vi "ReadOrSaveCases.vi"(9 "Location":enum16{"CUMC", "SERI", "VMR", "Aline", "UTEX"}(ring)=enum."SERI", 10 "New Case":T1, 11 "Save(T)\\Read(F)":bool) -> (2 "Case List":string[](array[string]), 3 "CaseArray":T2(array[cluster]))   [LabVIEW 2022 SP3]
uses:
  ScanningControl/Digitizers/-DigitizerRoutines/Digitizer.ctl
panel:
  out "path":path
  in  "Acquistion Parameters":T3={"Sampling Rate"=250.0, "Ref Delay (ms)"=0.0, "rf points per line"=2048, "rf lines"=256, "Dig Scale"=4.0} {"Dig Scale" items=["5 V"=5.0, "2 V"=2.0, "1 V"=1.0, "500 mV"=0.5, "200 mV"=0.2, "100 mV"=0.1, "50 mV"=0.05]; "rf lines" min=1; "rf points per line" min=1; "Ref Delay (ms)" format="%.2f"}
  in  "Sector?":bool=TRUE
  in  "Filter Prams":T4={"low cutoff"=20, "order"=81, "high cutoff"=60}
  in  "Timeout (s)":dbl=0.15
  in  "Probe":T5(ring)
  in  "Scan Info":T6
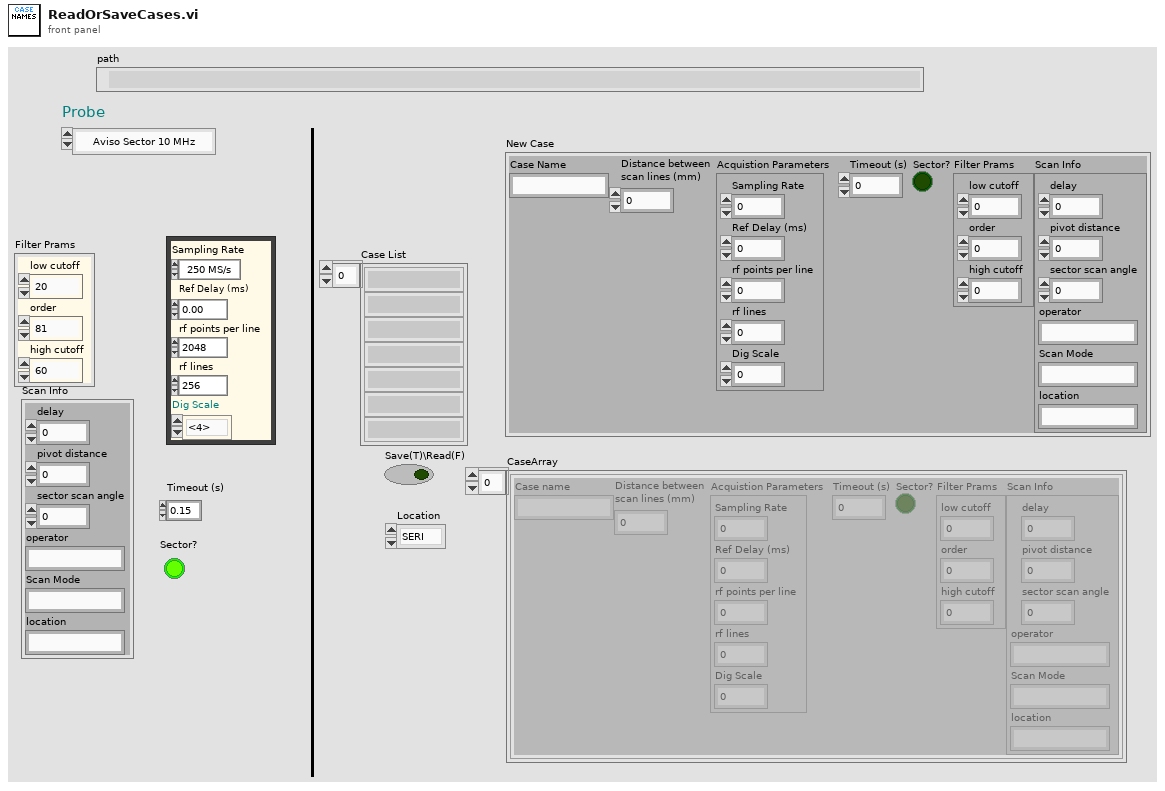
[diagram p1: front panel]
types:
  T1 = cluster{"Case Name":string, "Distance between\nscan lines (mm)":sgl, "Acquistion Parameters":cluster{"Sampling Rate":dbl, "Ref Delay (ms)":dbl, "rf points per line":i32, "rf lines":i32, "Dig Scale":dbl}, "Timeout (s)":dbl, "Sector?":bool, "Filter Prams":cluster{"low cutoff":i32, "order":i32, "high cutoff":i32}, "Scan Info":cluster{"delay":sgl, "pivot distance":sgl, "sector scan angle":sgl, "operator":string, "Scan Mode":string, "location":string}}
  T2 = cluster{"Case name":string, "Distance between\nscan lines (mm)":sgl, "Acquistion Parameters":cluster{"Sampling Rate":dbl, "Ref Delay (ms)":dbl, "rf points per line":i32, "rf lines":i32, "Dig Scale":dbl}, "Timeout (s)":dbl, "Sector?":bool, "Filter Prams":cluster{"low cutoff":i32, "order":i32, "high cutoff":i32}, "Scan Info":cluster{"delay":sgl, "pivot distance":sgl, "sector scan angle":sgl, "operator":string, "Scan Mode":string, "location":string}}[]
  T3 = cluster{"Sampling Rate":dbl, "Ref Delay (ms)":dbl, "rf points per line":i32, "rf lines":i32, "Dig Scale":dbl}
  T4 = cluster{"low cutoff":i32, "order":i32, "high cutoff":i32}
  T5 = enum16{"Aviso Sector 10 MHz", "Aviso Sector 20 MHz Retina", "Aviso Sector 20 MHz", "Aviso Lin50", "UTEX 50MHz", "Custom"}
  T6 = cluster{"delay":sgl, "pivot distance":sgl, "sector scan angle":sgl, "operator":string, "Scan Mode":string, "location":string}
  T7 = typedef "Digitizer.ctl" = enum16{"Acqiris Digitizer", "NI Digitizer", "LeCroy", "GaGe", "AlazarTech", "No Digitizer", "Teledyne"}
  T8 = enum16{"open", "replace", "create", "open or create", "replace or create", "replace or create with confirmation"}
  T9 = cluster{"Case Name":string, "Distance between\nscan lines (mm)":sgl, "Acquistion Parameters":cluster{"Sampling Rate":dbl, "Ref Delay (ms)":dbl, "rf points per line":i32, "rf lines":i32, "Dig Scale":dbl}, "Timeout (s)":dbl, "Sector?":bool, "Filter Prams":cluster{"low cutoff":i32, "order":i32, "high cutoff":i32}, "Scan Info":cluster{"delay":sgl, "pivot distance":sgl, "sector scan angle":sgl, "operator":string, "Scan Mode":string, "location":string}}[]
  T10 = cluster{"Sampling Rate":dbl, "Ref Delay (ms)":dbl, "rf points per line":i32, "rf lines":i32, "Voltage Scale 1":dbl}
  T11 = enum16{"Aviso Sector 10 MHz", "Aviso Sector 20 MHz Retina", "Aviso Sector 20 MHz", "Aviso Lin50", "Custom"}
  T12 = cluster{string, "Distance between\nscan lines (mm)":sgl, "Acquistion Parameters":cluster{"Sampling Rate":dbl, "Ref Delay (ms)":dbl, "rf points per line":i32, "rf lines":i32, "Dig Scale":dbl}, "Timeout (s)":dbl, "Sector?":bool, "Filter Prams":cluster{"low cutoff":i32, "order":i32, "high cutoff":i32}, "Scan Info":cluster{"delay":sgl, "pivot distance":sgl, "sector scan angle":sgl, "operator":string, "Scan Mode":string, "location":string}}
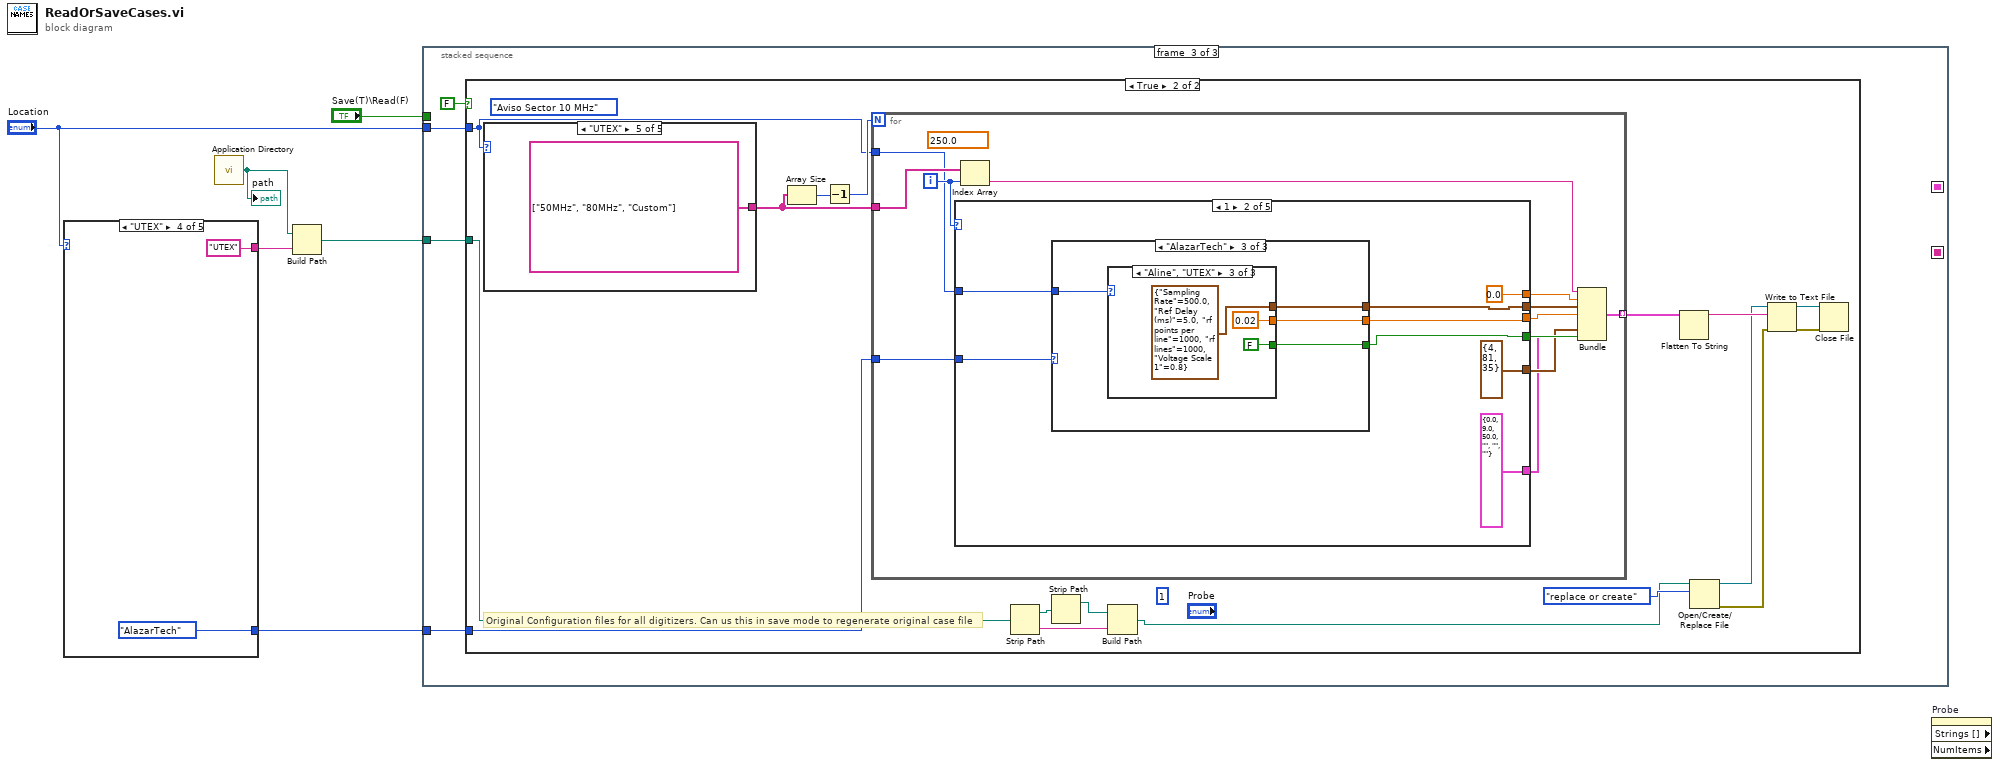
[diagram p0: block diagram]
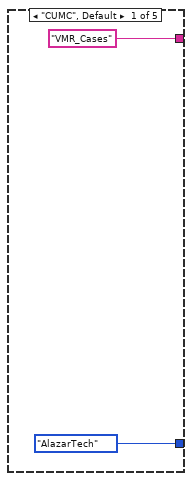
[diagram p2: hidden frame]
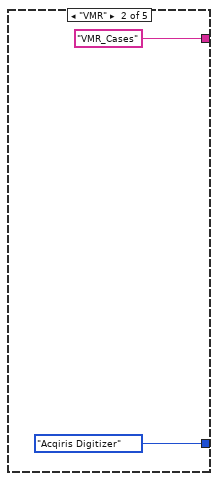
[diagram p3: hidden frame]
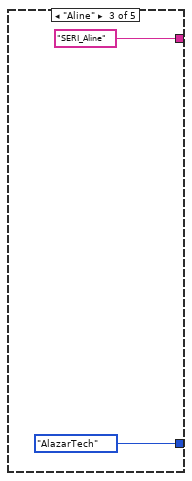
[diagram p4: hidden frame]
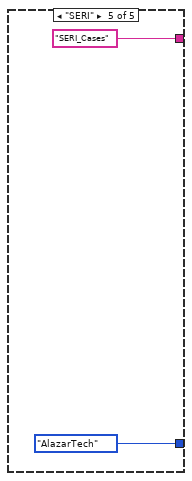
[diagram p5: hidden frame]
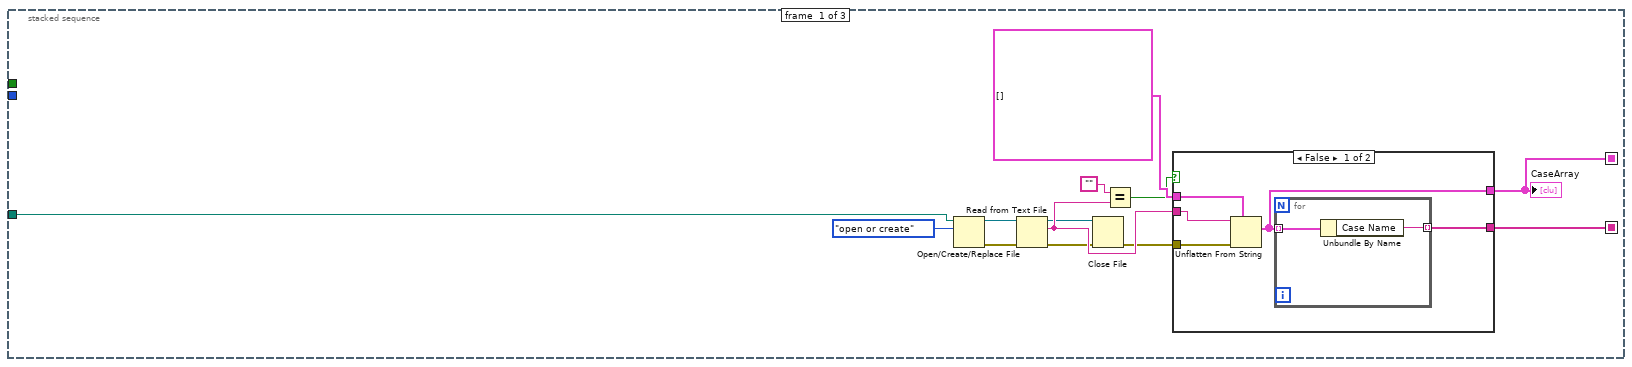
[diagram p6: hidden frame]
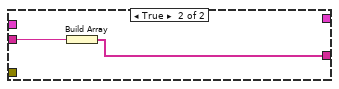
[diagram p7: hidden frame]
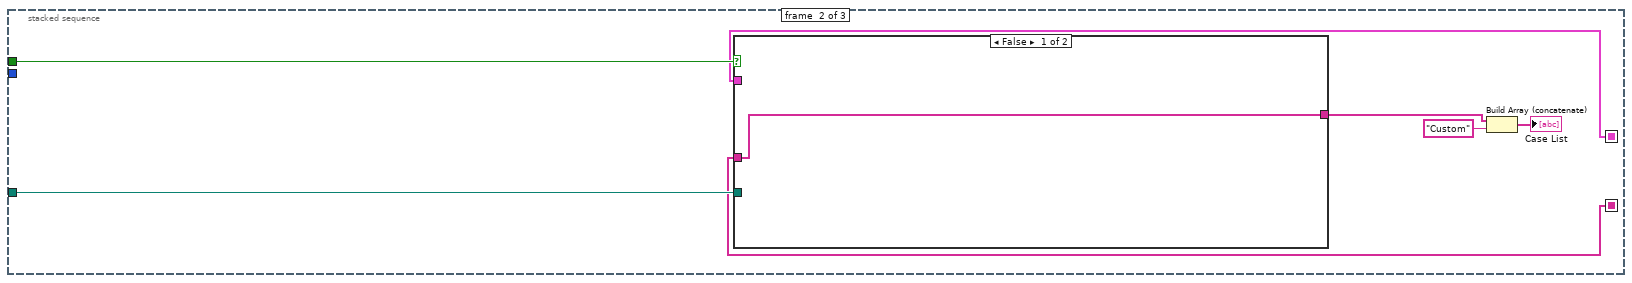
[diagram p8: hidden frame]
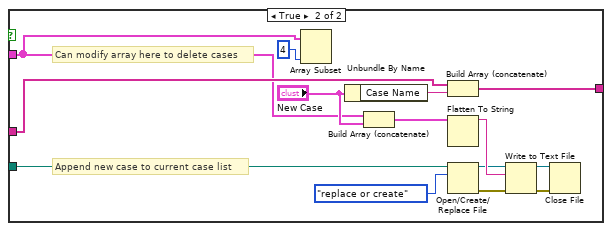
[diagram p9: hidden frame]
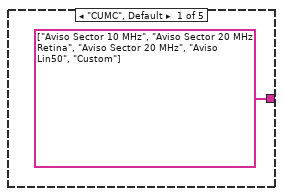
[diagram p11: hidden frame]
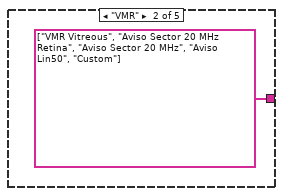
[diagram p12: hidden frame]
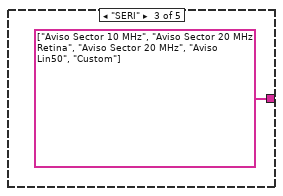
[diagram p13: hidden frame]
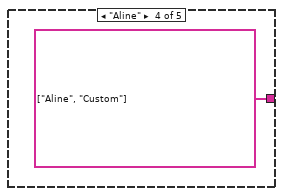
[diagram p14: hidden frame]
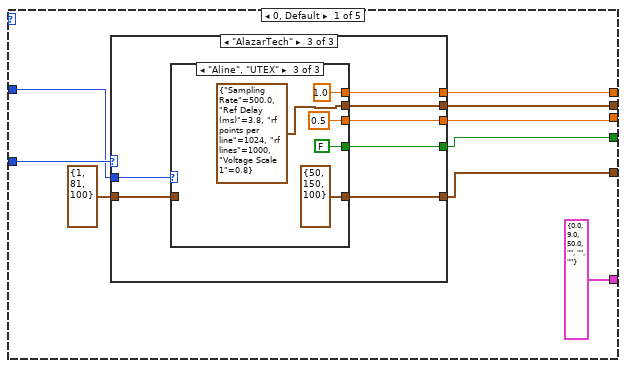
[diagram p15: hidden frame]
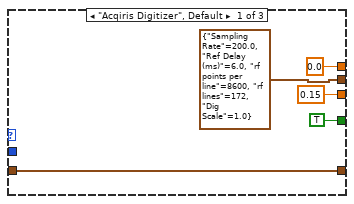
[diagram p16: hidden frame]
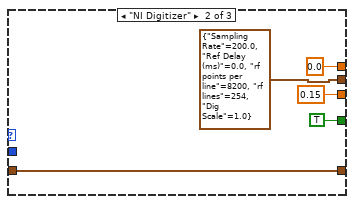
[diagram p17: hidden frame]
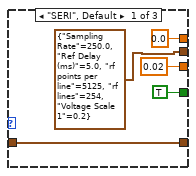
[diagram p18: hidden frame]
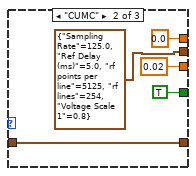
[diagram p19: hidden frame]
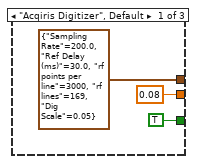
[diagram p20: hidden frame]
diagram:
  n1 = case shown="\"UTEX\"" "Location" {
    tunnel: ["VMR_Cases" "VMR_Cases" "SERI_Aline" "UTEX" "SERI_Cases"] -> w4
    tunnel: [Digitizer."AlazarTech" ("Main Digitizer") Digitizer."Acqiris Digitizer" ("Main Digitizer") Digitizer."AlazarTech" ("Main Digitizer") Digitizer."AlazarTech" ("Main Digitizer") Digitizer."AlazarTech" ("Main Digitizer")] -> w1
    frame "CUMC", Default {
    }
    frame "VMR" {
    }
    frame "Aline" {
    }
    frame "UTEX" {
    }
    frame "SERI" {
    }
  }
  n2 = call <vilib>:"Application Directory.vi"() -> ("Application Directory"=w3:path)
  "path" <- w3
  n3 = Build Path(base path=w3, name or relative path=w4) -> (appended path=w5:path)
  n4 = stacked-sequence {
    seq-local: [w18 _ _] -> [_ w44 _]
    seq-local: [w17 _ _] -> [_ w42 _]
    tunnel: w5 -> [w28 w43 w64]
    tunnel: "Save(T)\\Read(F)" -> [_ w45 _]
    tunnel: "Location" -> [_ _ w63]
    tunnel: w1 -> [_ _ w61]
    frame #0 {
      n5 = Open/Create/Replace File(file path (use dialog)=w28, operation (0:open)=T8."open or create") -> (refnum out=w27:refnum<file>, error out=w26:errorcluster)  [unwired: 4 in, 1 out]
      n6 = Read from Text File(file (use dialog)=w27, error in=w26) -> (refnum out=w19:refnum<file>, text=w23:string, error out=w21:errorcluster)  [unwired: 2 in, 1 out]
      n7 = Close File(refnum=w19, error in=w21) -> (error out=w20:errorcluster)  [unwired: 1 out]
      n8 = Equal?(x="", y=w23) -> (x = y?=w22:bool)
      n9 = case shown="False" w22 {
        tunnel: T9 [] -> [w34 _]
        tunnel: w20 -> [w33 _]
        tunnel: w23 -> [w32 w38]
        tunnel: [w31 w37] -> w17
        tunnel: [w30 _] -> w18
        frame False {
          n10 = Unflatten From String(type=w34, binary string=w32, error in (no error)=w33) -> (value=w30:T9)  [unwired: 2 in, 2 out]
          n11 = for {
            tunnel: w30 -> [w36] mode=indexing
            tunnel: [w35] -> w31 mode=indexing
            n12 = Unbundle By Name(w36) -> ("Case Name"=w35:string)
          }
        }
        frame True {
          n13 = Build Array(w38) -> (w37:string[])
        }
      }
      "CaseArray" <- w18
    }
    frame #1 {
      n14 = case shown="False" w45 {
        tunnel: w44 -> [_ w49]
        tunnel: w43 -> [_ w54]
        tunnel: w42 -> [w46 w52]
        tunnel: [w46 w50] -> w41
        frame False {
        }
        frame True {
          # "Can modify array here to delete cases"
          # "Append new case to current case list"
          n15 = Array Subset(array=w49, length=4) -> ()  [unwired: 1 in, 1 out]
          n16 = Unbundle By Name("New Case") -> ("Case Name"=w51:string)
          n17 = Build Array (concatenate)(w49, "New Case") -> (w47:T9)
          n18 = Build Array (concatenate)(w52, w51) -> (w50:string[])
          n19 = Flatten To String(anything=w47) -> (data string=w60:string)  [unwired: 3 in, 2 out]
          n20 = Open/Create/Replace File(file path (use dialog)=w54, operation (0:open)=T8."replace or create") -> (refnum out=w56:refnum<file>, error out=w57:errorcluster)  [unwired: 4 in, 1 out]
          n21 = Write to Text File(file (use dialog)=w56, text=w60, error in=w57) -> (refnum out=w59:refnum<file>, error out=w58:errorcluster)  [unwired: 1 in, 1 out]
          n22 = Close File(refnum=w59, error in=w58) -> ()  [unwired: 2 out]
        }
      }
      n23 = Build Array (concatenate)(w41, "Custom" ("Case Name")) -> (→"Case List":string[])
    }
    frame #2 {
      n24 = case shown="True" FALSE {
        tunnel: w64 -> [_ w69]
        tunnel: w63 -> [_ w73]
        tunnel: w61 -> [_ w70]
        frame False {
        }
        frame True {
          (unwired) 1
          (unwired) T11."Aviso Sector 10 MHz" ("Probe")
          # "Original Configuration files for all digitizers. Can us this in save mode to regenerate original case file"
          n25 = case shown="\"UTEX\"" w73 {
            tunnel: [string[] ["Aviso Sector 10 MHz", "Aviso Sector 20 MHz Retina", "Aviso Sector 20 MHz", "Aviso Lin50", "Custom"] ("Strings []") string[] ["VMR Vitreous", "Aviso Sector 20 MHz Retina", "Aviso Sector 20 MHz", "Aviso Lin50", "Custom"] ("Strings []") string[] ["Aviso Sector 10 MHz", "Aviso Sector 20 MHz Retina", "Aviso Sector 20 MHz", "Aviso Lin50", "Custom"] ("Strings []") string[] ["Aline", "Custom"] ("Strings []") string[] ["50MHz", "80MHz", "Custom"] ("Strings []")] -> w72
            frame "CUMC", Default {
            }
            frame "VMR" {
            }
            frame "SERI" {
            }
            frame "Aline" {
            }
            frame "UTEX" {
            }
          }
          n26 = Array Size(array=w72) -> (size(s)=w71:i32)
          n27 = Decrement(x=w71) -> (x-1=w74:i32)
          n28 = for {
            N: w74 -> [_]
            tunnel: w72 -> [w89]
            tunnel: [w91] -> w79 mode=indexing
            tunnel: w73 -> [w88]
            tunnel: w70 -> [w87]
            i -> [w90]
            (unwired) 250.0 ("Sampling Rate")
            n29 = case shown="1" w90 {
              tunnel: [w101 sgl 0.0 sgl 0.0 sgl 50.0 sgl 0.0 ("Distance between\nscan lines (mm)")] -> w98
              tunnel: [w107 w146 w173 w191 "Acquistion Parameters"] -> w97
              tunnel: [w99 T4 {"low cutoff"=4, "order"=81, "high cutoff"=35} ("Filter Prams") T4 {"low cutoff"=4, "order"=81, "high cutoff"=35} ("Filter Prams") T4 {"low cutoff"=20, "order"=81, "high cutoff"=60} ("Filter Prams") "Filter Prams"] -> w94
              tunnel: [T6 {"delay"=0.0, "pivot distance"=9.0, "sector scan angle"=50.0, "operator"="", "Scan Mode"="", "location"=""} ("Scan Info") T6 {"delay"=0.0, "pivot distance"=9.0, "sector scan angle"=50.0, "operator"="", "Scan Mode"="", "location"=""} ("Scan Info") T6 {"delay"=0.0, "pivot distance"=9.0, "sector scan angle"=50.0, "operator"="", "Scan Mode"="", "location"=""} ("Scan Info") T6 {"delay"=0.0, "pivot distance"=0.0, "sector scan angle"=0.0, "operator"="", "Scan Mode"="", "location"=""} ("Scan Info") "Scan Info"] -> w93
              tunnel: w87 -> [w105 w143 w170 w192 _]
              tunnel: [w104 w142 w169 w190 "Timeout (s)"] -> w96
              tunnel: [w102 w140 TRUE FALSE "Sector?"] -> w95
              tunnel: w88 -> [w103 w141 w167 w188 _]
              frame 0, Default {
                n30 = case shown="\"AlazarTech\"" w105 {
                  tunnel: [T3 {"Sampling Rate"=200.0, "Ref Delay (ms)"=6.0, "rf points per line"=8600, "rf lines"=172, "Dig Scale"=1.0} ("Acquistion Parameters") T3 {"Sampling Rate"=200.0, "Ref Delay (ms)"=0.0, "rf points per line"=8200, "rf lines"=254, "Dig Scale"=1.0} ("RF data Sampling") w124] -> w107
                  tunnel: [0.15 ("Timeout (s)") 0.15 ("Timeout (s)") w123] -> w104
                  tunnel: w103 -> [_ _ w122]
                  tunnel: [TRUE TRUE w121] -> w102
                  tunnel: [sgl 0.0 sgl 0.0 w120] -> w101
                  tunnel: [w108 w113 w119] -> w99
                  tunnel: T4 {"low cutoff"=1, "order"=81, "high cutoff"=100} ("Filter Prams") -> [w108 w113 w118]
                  frame "Acqiris Digitizer", Default {
                  }
                  frame "NI Digitizer" {
                  }
                  frame "AlazarTech" {
                    n31 = case shown="\"Aline\", \"UTEX\"" w122 {
                      tunnel: [T10 {"Sampling Rate"=250.0, "Ref Delay (ms)"=5.0, "rf points per line"=5125, "rf lines"=254, "Voltage Scale 1"=0.2} ("RF data Sampling") T10 {"Sampling Rate"=125.0, "Ref Delay (ms)"=5.0, "rf points per line"=5125, "rf lines"=254, "Voltage Scale 1"=0.8} ("RF data Sampling") T10 {"Sampling Rate"=500.0, "Ref Delay (ms)"=3.8, "rf points per line"=1024, "rf lines"=1000, "Voltage Scale 1"=0.8} ("RF data Sampling")] -> w124
                      tunnel: [0.02 ("Timeout (s)") 0.02 ("Timeout (s)") 0.5 ("Timeout (s)")] -> w123
                      tunnel: [TRUE TRUE FALSE] -> w121
                      tunnel: [sgl 0.0 sgl 0.0 sgl 1.0] -> w120
                      tunnel: [w125 w130 T4 {"low cutoff"=50, "order"=150, "high cutoff"=100} ("Filter Prams")] -> w119
                      tunnel: w118 -> [w125 w130 _]
                      frame "SERI", Default {
                      }
                      frame "CUMC" {
                      }
                      frame "Aline", "UTEX" {
                      }
                    }
                  }
                }
              }
              frame 1 {
                n32 = case shown="\"AlazarTech\"" w143 {
                  tunnel: [T3 {"Sampling Rate"=200.0, "Ref Delay (ms)"=30.0, "rf points per line"=3000, "rf lines"=169, "Dig Scale"=0.05} ("Acquistion Parameters") T3 {"Sampling Rate"=200.0, "Ref Delay (ms)"=0.0, "rf points per line"=8200, "rf lines"=254, "Dig Scale"=1.0} ("RF data Sampling") w157] -> w146
                  tunnel: [0.08 ("Timeout (s)") 0.15 ("Timeout (s)") w156] -> w142
                  tunnel: w141 -> [_ _ w155]
                  tunnel: [TRUE TRUE w154] -> w140
                  frame "Acqiris Digitizer", Default {
                  }
                  frame "NI Digitizer" {
                  }
                  frame "AlazarTech" {
                    n33 = case shown="\"Aline\", \"UTEX\"" w155 {
                      tunnel: [T10 {"Sampling Rate"=250.0, "Ref Delay (ms)"=5.0, "rf points per line"=5125, "rf lines"=254, "Voltage Scale 1"=0.2} ("RF data Sampling") T10 {"Sampling Rate"=125.0, "Ref Delay (ms)"=30.0, "rf points per line"=3000, "rf lines"=254, "Voltage Scale 1"=0.8} ("RF data Sampling") T10 {"Sampling Rate"=500.0, "Ref Delay (ms)"=5.0, "rf points per line"=1000, "rf lines"=1000, "Voltage Scale 1"=0.8} ("RF data Sampling")] -> w157
                      tunnel: [0.02 ("Timeout (s)") 0.02 ("Timeout (s)") 0.02 ("Timeout (s)")] -> w156
                      tunnel: [TRUE TRUE FALSE] -> w154
                      frame "SERI", Default {
                      }
                      frame "CUMC" {
                      }
                      frame "Aline", "UTEX" {
                      }
                    }
                  }
                }
              }
              frame 2 {
                n34 = case shown="\"AlazarTech\"" w170 {
                  tunnel: [T3 {"Sampling Rate"=200.0, "Ref Delay (ms)"=5.0, "rf points per line"=8000, "rf lines"=168, "Dig Scale"=0.05} ("Acquistion Parameters") T3 {"Sampling Rate"=250.0, "Ref Delay (ms)"=5.0, "rf points per line"=10250, "rf lines"=254, "Dig Scale"=1.0} ("RF data Sampling") w181] -> w173
                  tunnel: [0.08 ("Timeout (s)") 0.15 ("Timeout (s)") w180] -> w169
                  tunnel: w167 -> [_ _ w179]
                  frame "Acqiris Digitizer", Default {
                  }
                  frame "NI Digitizer" {
                  }
                  frame "AlazarTech" {
                    n35 = case shown="\"UTEX\"" w179 {
                      tunnel: [T10 {"Sampling Rate"=250.0, "Ref Delay (ms)"=5.0, "rf points per line"=5125, "rf lines"=254, "Voltage Scale 1"=0.2} ("RF data Sampling") T10 {"Sampling Rate"=500.0, "Ref Delay (ms)"=2.468, "rf points per line"=650, "rf lines"=254, "Voltage Scale 1"=0.2} ("RF data Sampling") T10 {"Sampling Rate"=125.0, "Ref Delay (ms)"=5.0, "rf points per line"=5125, "rf lines"=254, "Voltage Scale 1"=0.4} ("RF data Sampling")] -> w181
                      tunnel: [0.02 ("Timeout (s)") 0.02 ("Timeout (s)") 0.02 ("Timeout (s)")] -> w180
                      frame "SERI", Default {
                      }
                      frame "UTEX" {
                      }
                      frame "CUMC" {
                      }
                    }
                  }
                }
              }
              frame 3 {
                n36 = case shown="\"NI Digitizer\"" w192 {
                  tunnel: [T3 {"Sampling Rate"=400.0, "Ref Delay (ms)"=5.4, "rf points per line"=8000, "rf lines"=254, "Dig Scale"=0.5} ("Acquistion Parameters") T3 {"Sampling Rate"=250.0, "Ref Delay (ms)"=5.4, "rf points per line"=5000, "rf lines"=254, "Dig Scale"=0.4} ("RF data Sampling") w202] -> w191
                  tunnel: [0.08 ("Timeout (s)") 0.15 ("Timeout (s)") w201] -> w190
                  tunnel: w188 -> [_ _ w200]
                  frame "Acqiris Digitizer", Default {
                  }
                  frame "NI Digitizer" {
                  }
                  frame "AlazarTech" {
                    n37 = case shown="\"SERI\", Default" w200 {
                      tunnel: [T10 {"Sampling Rate"=250.0, "Ref Delay (ms)"=5.0, "rf points per line"=5125, "rf lines"=254, "Voltage Scale 1"=0.2} ("RF data Sampling") T10 {"Sampling Rate"=125.0, "Ref Delay (ms)"=5.4, "rf points per line"=2500, "rf lines"=254, "Voltage Scale 1"=0.8} ("RF data Sampling")] -> w202
                      tunnel: [0.02 ("Timeout (s)") 0.02 ("Timeout (s)")] -> w201
                      frame "SERI", Default {
                      }
                      frame "CUMC" {
                      }
                    }
                  }
                }
              }
              frame 4 {
              }
            }
            n38 = Index Array(array=w89, index=w90) -> (element=w92:string)
            n39 = Bundle(w92, "Distance between\nscan lines (mm)"=w98, "Acquistion Parameters"=w97, "Timeout (s)"=w96, "Sector?"=w95, "Filter Prams"=w94, "Scan Info"=w93) -> (w91:T12)  [unwired: 1 in]
          }
          n40 = Strip Path(path=w69) -> (stripped path=w68:path, name=w66:string)
          n41 = Strip Path(path=w68) -> (stripped path=w67:path)  [unwired: 1 out]
          n42 = Build Path(base path=w67, name or relative path=w66) -> (appended path=w65:path)
          n43 = Flatten To String(anything=w79) -> (data string=w81:string)  [unwired: 3 in, 2 out]
          n44 = Open/Create/Replace File(file path (use dialog)=w65, operation (0:open)=T8."replace or create") -> (refnum out=w76:refnum<file>, error out=w77:errorcluster)  [unwired: 4 in, 1 out]
          n45 = Write to Text File(file (use dialog)=w76, text=w81, error in=w77) -> (refnum out=w80:refnum<file>, error out=w78:errorcluster)  [unwired: 1 in, 1 out]
          n46 = Close File(refnum=w80, error in=w78) -> ()  [unwired: 2 out]
        }
      }
    }
  }
  n47 = property on="Probe" class="Enum (strict)" props=["Strings []", "NumItems"]() -> ()  [unwired: 2 in, 4 out]
